vi "Update Function List.vi"(8 "error in (no error)":errorcluster, 10 "List of Functions":string[](array[string]), 11 "Operator UI in":refnum<class "Controller UI.lvclass">) -> (0 "error out":errorcluster, 3 "Operator UI out":refnum<class "Controller UI.lvclass">)   [LabVIEW 2016, in "Controller UI.lvlib" / "Controller UI.lvclass"]
uses:
  <userlib>/Common Components/Controller UI/Controller UI.lvclass
  <userlib>/Common Components/Controller UI/Controller UI.lvclass/Controller UI.ctl
  <userlib>/Common Components/Controller UI/Accessors/Read Function.vi
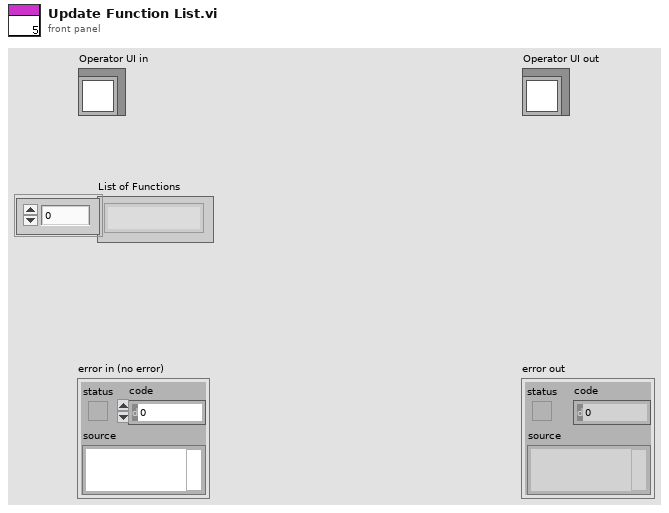
[diagram p1: front panel]
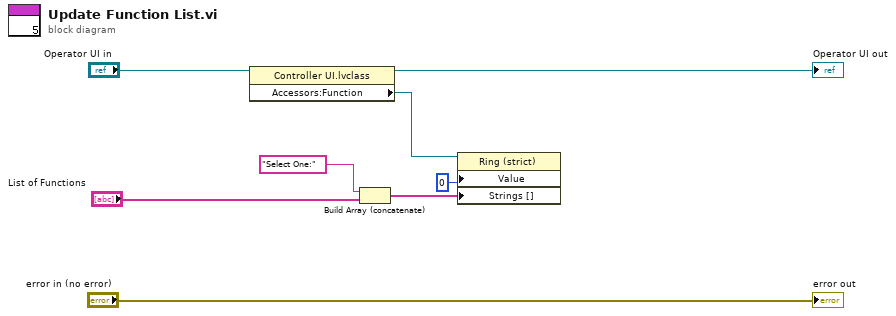
[diagram p0: block diagram]
diagram:
  n1 = property class="Controller UI.lvclass"(reference="Operator UI in") -> (reference out=→"Operator UI out":refnum<class "Controller UI.lvclass">, "Accessors:Function"=w1:refnum<vi>)  [unwired: 1 in, 1 out]
  n2 = Build Array (concatenate)("Select One:", "List of Functions") -> (w5:string[])
  n3 = property class="Ring (strict)"(reference=w1, "Value"=u16 0, "Strings []"=w5) -> ()  [unwired: 1 in, 2 out]
  "error out" <- "error in (no error)"
